vi "Cryo-Con Get H.vi"(8 "error in (no error)":errorcluster, 11 "VISA Resource Name":refnum<visa-resource-name>) -> (0 "error out":errorcluster, 1 "data string":string, 3 "VISA Resource Name Out":refnum<visa-resource-name>, 4 "Heat %":dbl format="%.2f")   [LabVIEW 2016]
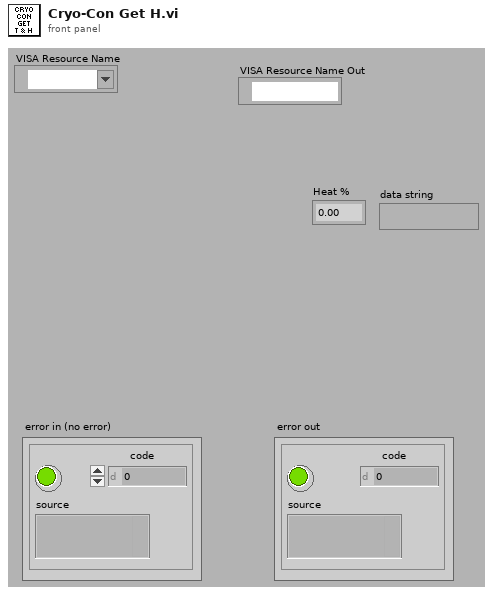
[diagram p1: front panel]
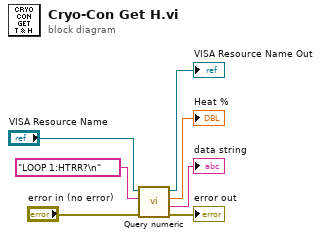
[diagram p0: block diagram]
diagram:
  n1 = call "Query numeric.vi"("Error In"="error in (no error)", "Query String"="LOOP 1:HTRR?\n", "VISA resource name"="VISA Resource Name") -> ("Error Out"=→"error out":errorcluster, "data string out"=→"data string":string, "Numeric"=→"Heat %":dbl, "VISA resource name out"=→"VISA Resource Name Out":refnum<visa-resource-name>)  [unwired: 5 in]
